vi "Display Module - Switch On and Off.vi"(0 "Image Refs":T1[](array[typedef]), 11 "IMAQ Display Refs":refnum<vi>[](array[refnum])) -> ()   [LabVIEW 2020]
uses:
  <vilib>/vision/Image Controls.llb/IMAQ Image.ctl
  <vilib>/Utility/miscctls.llb/LVPointTypeDef.ctl
panel:
  in  "Quit":bool
  # "Click on a display to change its state."
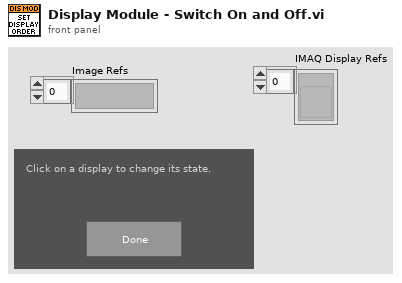
[diagram p1: front panel]
types:
  T1 = typedef "IMAQ Image.ctl" = refnum<image>
  T2 = enum16{"Always On", "Always Off", "Off While Running"}
  T3 = typedef "LVPointTypeDef.ctl" = cluster{"Horizontal":i16, "Vertical":i16}
  T4 = enum16{"User-specified Font", "Application Font", "System Font", "Dialog Font"}
  T5 = cluster{"Desired Font (Application)":enum16{"User-specified Font", "Application Font", "System Font", "Dialog Font"}, "[User-specified Font]":cluster{"Font Name":string, "Size":i16, "Strikeout?":bool, "Italic?":bool, "Underline?":bool, "Outline?":bool, "Shadow?":bool, "Bold?":bool, "Rotation Angle":dbl}, "Horizontal Alignment":i16, "Vertical Alignment":i16}
  T6 = cluster{"Font Name":string, "Size":i16, "Strikeout?":bool, "Italic?":bool, "Underline?":bool, "Outline?":bool, "Shadow?":bool, "Bold?":bool, "Rotation Angle":dbl}
  T7 = typedef "LVRectTypeDef.ctl" = cluster{"Left":i16, "Top":i16, "Right":i16, "Bottom":i16}
  T8 = typedef "LVBoundsTypeDef.ctl" = cluster{"Width":u32, "Height":u32}
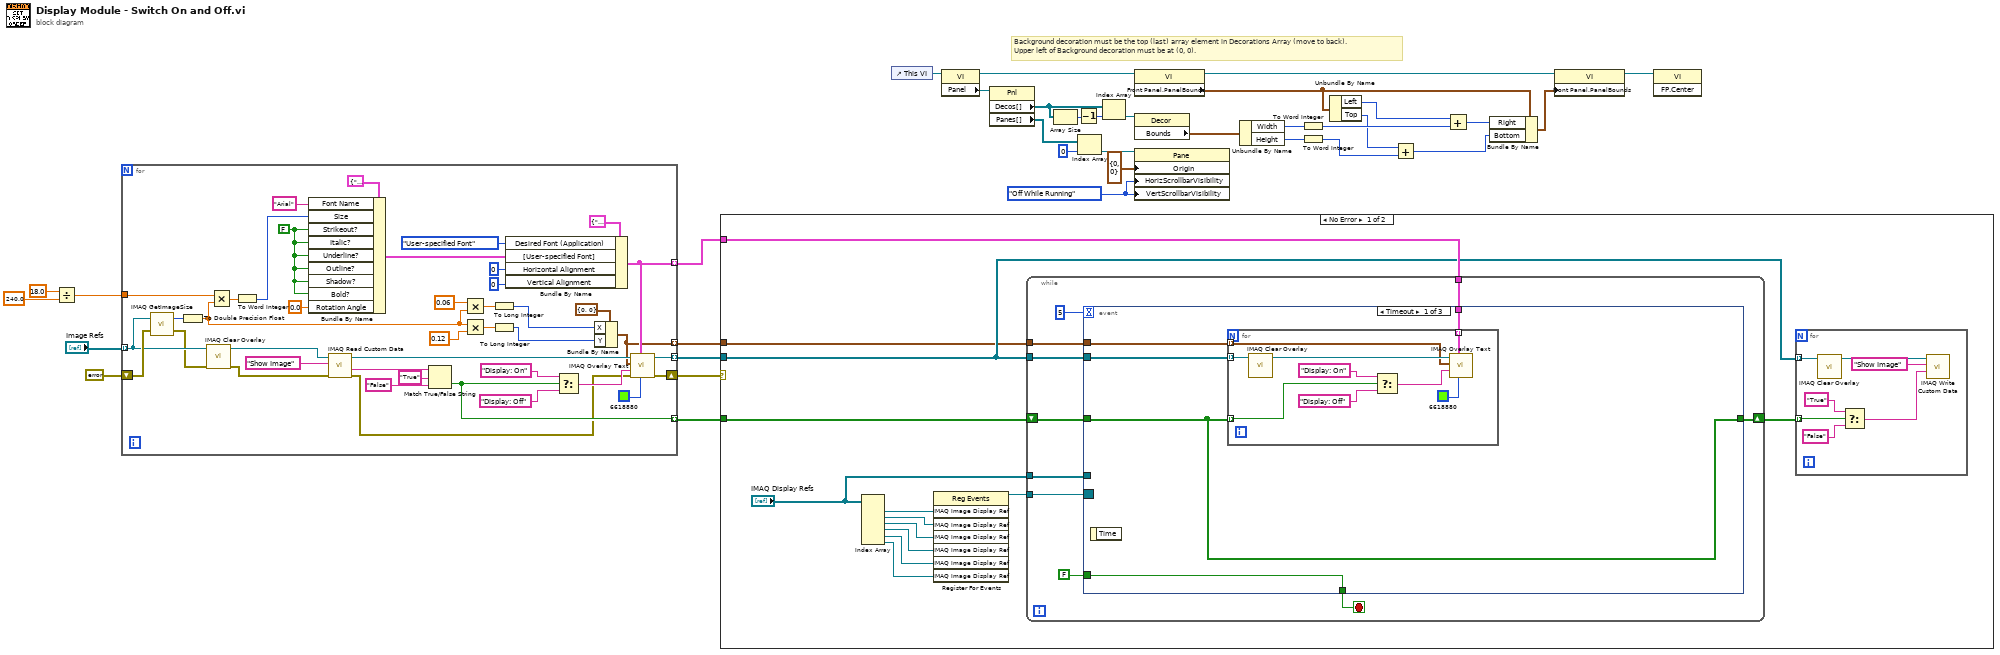
[diagram p0: block diagram]
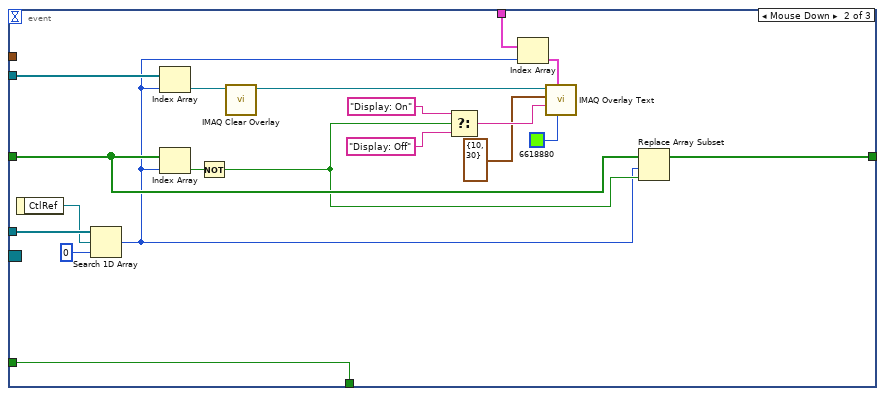
[diagram p2: hidden frame]
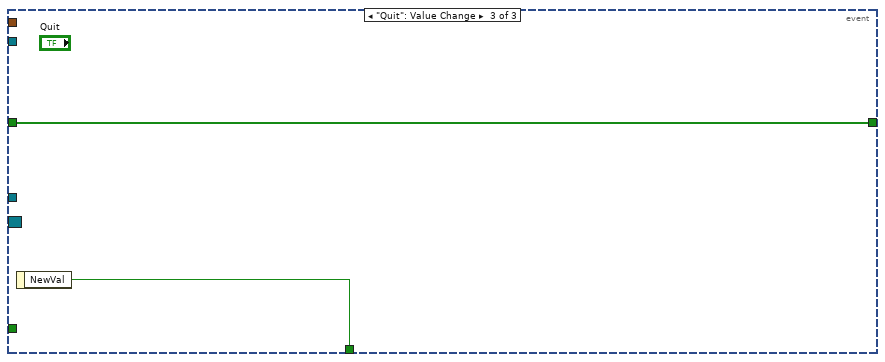
[diagram p3: hidden frame]
diagram:
  w22 = T2."Off While Running" ("Vertical Scrollbar Visibility")
  # "Background decoration must be the top (last) array element in Decorations Array (move to back).\nUpper left of Background decoration must be at (0, 0)."
  n1 = Divide(x=18.0, y=240.0) -> (x/y=w2:dbl)
  n2 = for {
    tunnel: "Image Refs" -> [w52] mode=indexing
    tunnel: [w67] -> w33 mode=indexing
    tunnel: [w66] -> w34 mode=indexing
    shift-right: [w63] -> w6
    shift-left: errorcluster {"status"=FALSE, "code"=0, "source"=""} ("error out") -> [w53]
    tunnel: w2 -> [w49]
    tunnel: [w47] -> w3 mode=indexing
    tunnel: [w41] -> w1 mode=indexing
    w59 = FALSE ("Strikeout?")
    n3 = call "IMAQ GetImageSize"("Image"=w52, "error in (no error)"=w53) -> ("Y Resolution"=w50:i32, "error out"=w51:errorcluster)  [unwired: 2 in, 1 out]
    n4 = To Double Precision Float(number=w50) -> (double precision float=w38:dbl)
    n5 = call "IMAQ Clear Overlay"("error in (no error)"=w51, "Image"=w52) -> ("error out"=w64:errorcluster, "Image Out"=w65:T1)  [unwired: 8 in]
    n6 = Multiply(x=w49, y=w38) -> (x*y=w44:dbl)
    n7 = To Word Integer(number=w44) -> (16bit integer=w46:i16)
    n8 = Bundle By Name(cluster=T6 {"Font Name"="", "Size"=0, "Strikeout?"=FALSE, "Italic?"=FALSE, "Underline?"=FALSE, "Outline?"=FALSE, "Shadow?"=FALSE, "Bold?"=FALSE, "Rotation Angle"=0.0} ("[User-specified Font]"), "Font Name"="Arial", "Size"=w46, "Strikeout?"=w59, "Italic?"=w59, "Underline?"=w59, "Outline?"=w59, "Shadow?"=w59, "Bold?"=w59, "Rotation Angle"=0.0) -> (w62:T6)
    n9 = call "IMAQ Read Custom Data"("error in (no error)"=w64, "Key"="Show Image", "Image"=w65) -> ("error out"=w48:errorcluster, "Custom Data Out"=w76:string, "Image (duplicate)"=w72:T1)  [unwired: 6 in]
    n10 = Match True/False String(2:"False" ("false string"), 3:"True" ("true string"), 4:w76) -> (0:w66:bool)  [unwired: 1 out]
    n11 = Multiply(x=0.06, y=w38) -> (x*y=w39:dbl)
    n12 = Multiply(x=w38, y=0.12) -> (x*y=w42:dbl)
    n13 = To Long Integer(number=w39) -> (32bit integer=w36:i32)
    n14 = To Long Integer(number=w42) -> (32bit integer=w40:i32)
    n15 = Bundle By Name(cluster=T5 {"Desired Font (Application)"=enum."Application Font", "[User-specified Font]"={"Font Name"="", "Size"=12, "Strikeout?"=FALSE, "Italic?"=FALSE, "Underline?"=FALSE, "Outline?"=FALSE, "Shadow?"=FALSE, "Bold?"=FALSE, "Rotation Angle"=0.0}, "Horizontal Alignment"=0, "Vertical Alignment"=0} ("Font, Size & Style"), "Desired Font (Application)"=T4."User-specified Font", "[User-specified Font]"=w62, "Horizontal Alignment"=i16 0, "Vertical Alignment"=i16 0) -> (w47:T5)
    n16 = Select(t="Display: On" ("false string"), s=w66, f="Display: Off" ("false string")) -> (s? t:f=w68:string)
    n17 = Bundle By Name(cluster=cluster{"X":i32, "Y":i32} {"X"=0, "Y"=0} ("Origin"), "X"=w36, "Y"=w40) -> (w41:cluster{"X":i32, "Y":i32})
    n18 = call "IMAQ Overlay Text"("Text Color (black)"=u32 6618880, "Font, Size & Style"=w47, "error in (no error)"=w48, "String"=w68, "Origin"=w41, "Image"=w72) -> ("error out"=w63:errorcluster, "Image Out"=w67:T1)  [unwired: 4 in]
  }
  n19 = case shown="No Error" w6 {
    tunnel: w34 -> [w82 _]
    tunnel: w3 -> [w80 _]
    tunnel: w33 -> [w79 _]
    tunnel: w1 -> [w77 _]
    frame No Error {
      n20 = Index Array(array="IMAQ Display Refs") -> (element #1=w85:refnum<vi>, element #2=w89:refnum<vi>, element #3=w86:refnum<vi>, element #4=w87:refnum<vi>, element #5=w88:refnum<vi>, element #6=w83:refnum<vi>)  [unwired: 6 in]
      n21 = register-events(w85, w89, w86, w87, w88, w83) -> (reference out=w84:refnum<event-registration>)  [unwired: 2 in, 1 out]
      n22 = while {
        tunnel: w84 -> [w103]
        shift-right: [w98] -> w78
        shift-left: w82 -> [w101]
        tunnel: "IMAQ Display Refs" -> [w100]
        tunnel: w80 -> [w99]
        tunnel: w79 -> [w102]
        tunnel: w77 -> [w97]
        stop <- w106 stop-if-true
        n23 = event shown="[0] Timeout" {
          selector: w103 -> [_ _ _]
          dyn-events: _ -> [_ _ _]
          timeout: 5 -> [_ _ _]
          tunnel: [w111 w139 w141] -> w106
          tunnel: FALSE -> [w111 w139 _]
          tunnel: w102 -> [w110 w129 _]
          tunnel: w101 -> [w108 w126 w140]
          tunnel: w100 -> [_ w138 _]
          tunnel: w99 -> [w109 w123 _]
          tunnel: [w108 w125 w140] -> w98
          tunnel: w97 -> [w107 _ _]
          event Timeout {
            n24 = event-data() -> ()  [unwired: 1 in, 1 out]
            n25 = for {
              tunnel: w110 -> [w114] mode=indexing
              tunnel: w109 -> [w115] mode=indexing
              tunnel: w108 -> [w113] mode=indexing
              tunnel: w107 -> [w112] mode=indexing
              n26 = call "IMAQ Clear Overlay"("Image"=w114) -> ("Image Out"=w116:T1)  [unwired: 9 in, 1 out]
              n27 = Select(t="Display: On" ("false string"), s=w113, f="Display: Off" ("false string")) -> (s? t:f=w117:string)
              n28 = call "IMAQ Overlay Text"("Text Color (black)"=u32 6618880, "Font, Size & Style"=w115, "String"=w117, "Origin"=w112, "Image"=w116) -> ()  [unwired: 5 in, 2 out]
            }
          }
          event Mouse Down {
            n29 = event-data() -> ("CtlRef"=w137:refnum<vi>)  [unwired: 1 in]
            n30 = Search 1D Array(1D array=w138, element=w137, start index (0)=0) -> (index of element=w121:i32)
            n31 = Index Array(array=w129, index=w121) -> (element=w128:T1)
            n32 = Index Array(array=w126, index=w121) -> (element=w135:bool)
            n33 = Not(x=w135) -> (.not. x?=w124:bool)
            n34 = call "IMAQ Clear Overlay"("Image"=w128) -> ("Image Out"=w127:T1)  [unwired: 9 in, 1 out]
            n35 = Select(t="Display: On" ("false string"), s=w124, f="Display: Off" ("false string")) -> (s? t:f=w131:string)
            n36 = Index Array(array=w123, index=w121) -> (element=w122:T5)
            n37 = call "IMAQ Overlay Text"("Text Color (black)"=u32 6618880, "Font, Size & Style"=w122, "String"=w131, "Origin"=cluster{"X":i32, "Y":i32} {"X"=10, "Y"=30}, "Image"=w127) -> ()  [unwired: 5 in, 2 out]
            n38 = Replace Array Subset(array=w126, new element=w124, index=w121) -> (w125:bool[])
          }
          event "Quit": Value Change {
            n39 = event-data() -> ("NewVal"=w141:bool)  [unwired: 1 in]
          }
        }
      }
      n40 = for {
        tunnel: w79 -> [w93] mode=indexing
        tunnel: w78 -> [w96] mode=indexing
        n41 = call "IMAQ Clear Overlay"("Image"=w93) -> ("Image Out"=w92:T1)  [unwired: 9 in, 1 out]
        n42 = Select(t="True", s=w96, f="False") -> (s? t:f=w90:string)
        n43 = call "IMAQ Write Custom Data"("Custom Data In"=w90, "Key"="Show Image", "Image"=w92) -> ()  [unwired: 7 in, 2 out]
      }
    }
    frame Error {
    }
  }
  n44 = control-ref of="This VI"() -> (w15:refnum<vi>)
  n45 = property class="VI"(reference=w15) -> (reference out=w23:refnum<vi>, "Panel"=w16:refnum<vi>)  [unwired: 1 in, 1 out]
  n46 = property class="Pnl"(reference=w16) -> ("Decos[]"=w14:refnum<vi>[], "Panes[]"=w19:refnum<vi>[])  [unwired: 1 in, 2 out]
  n47 = Array Size(array=w14) -> (size(s)=w12:i32)
  n48 = Decrement(x=w12) -> (x-1=w13:i32)
  n49 = Index Array(array=w19, index=0) -> (element=w18:refnum<vi>)
  n50 = Index Array(array=w14, index=w13) -> (element=w21:refnum<vi>)
  n51 = property class="VI"(reference=w23) -> (reference out=w25:refnum<vi>, "Front Panel.PanelBounds"=w26:T7)  [unwired: 1 in, 1 out]
  n52 = property class="Decor"(reference=w21) -> ("Bounds"=w24:T8)  [unwired: 1 in, 2 out]
  n53 = property class="Pane"(reference=w18, "Origin"=T3 {"Horizontal"=0, "Vertical"=0}, "HorizScrollbarVisibility"=w22, "VertScrollbarVisibility"=w22) -> ()  [unwired: 1 in, 2 out]
  n54 = Unbundle By Name(w24) -> ("Width"=w29:u32, "Height"=w32:u32)
  n55 = To Word Integer(number=w29) -> (16bit integer=w31:i16)
  n56 = To Word Integer(number=w32) -> (16bit integer=w10:i16)
  n57 = Unbundle By Name(w26) -> ("Left"=w28:i16, "Top"=w11:i16)
  n58 = Add(x=w11, y=w10) -> (x+y=w9:i16)
  n59 = Add(x=w28, y=w31) -> (x+y=w30:i16)
  n60 = Bundle By Name(cluster=w26, "Right"=w30, "Bottom"=w9) -> (w27:T7)
  n61 = property class="VI"(reference=w25, "Front Panel.PanelBounds"=w27) -> (reference out=w8:refnum<vi>)  [unwired: 1 in, 1 out]
  n62 = invoke class="VI" method="FP.Center"(reference=w8) -> ()  [unwired: 2 in, 3 out]
